vi "TRIG_CHAN_AUX_OPOL.vi"(0 "VISA IN":refnum<visa-resource-name>, 1 "Aux":i32, 2 "Polarity":string(combo)="POS", 5 "error in":errorcluster, 7 "Channel":i32) -> (14 "VISA Out":refnum<visa-resource-name>, 19 "error out":errorcluster)   [LabVIEW 2018, in "PNA-X.lvlib"]
doc: "TRIGger:CHANnel<ch>:AUX<n>:OPOLarity <char> \n(Read-Write) Specifies the polarity of the Aux Output signal being supplied by the PNA. \nParameters \n<ch> Any existing channel number. If unspecified, value is set to 1. \n<n> Rear panel connector used to send or receive signals. \nPNA-X - choose from 1 (AUX TRIG 1) or 2 (AUX TRIG 2) \nAll other models: choose 1. (BNC Trig I/O \nIf unspecified, value is set to 1. \n<char> Choose from: \nPOSitive PNA sends positive going pulse. \nNEGative PNA sends negative going pulse. \nExamples TRIG:CHAN:AUX:OPOL NEG \ntrigger:channel2:aux2:opolarity positive \nQuery Syntax TRIGger:CHANnel<ch>:AUX<n>:OPOLarity? \nReturn Type Character \nDefault NEGative"
uses:
  PNA-X.lvlib
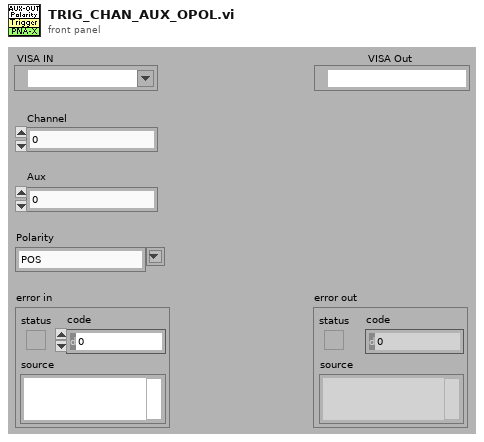
[diagram p1: front panel]
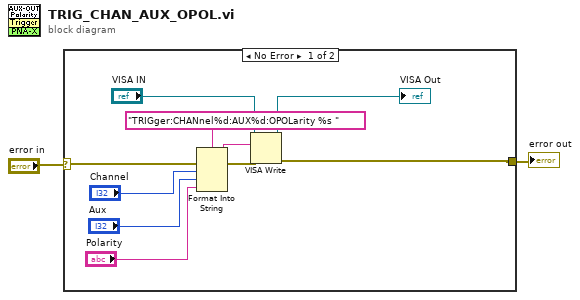
[diagram p0: block diagram]
diagram:
  n1 = case shown="No Error" "error in" {
    selector: "error in" -> [w12 w13]
    tunnel: [w7 w13] -> w1
    frame No Error {
      n2 = Format Into String(format string="TRIGger:CHANnel%d:AUX%d:OPOLarity %s " ("Cmdline"), error in=w12, "Channel", "Aux", "Polarity") -> (resulting string=w10:string, error out=w11:errorcluster)  [unwired: 1 in]
      n3 = VISA Write(VISA resource name="VISA IN", write buffer=w10, error in (no error)=w11) -> (VISA resource name out=→"VISA Out":refnum<visa-resource-name>, error out=w7:errorcluster)  [unwired: 1 out]
    }
    frame Error {
    }
  }
  "error out" <- w1
